vi "Custom Transient Response for Setpoints.vi"() -> (3 "SourceAdapt Parameters":T1 {"Current compensation frequency" scale=50.0..1000000.0 scale format="%#_6pHz"; "Voltage compensation frequency" scale=50.0..1000000.0 scale format="%#_6pHz"; "Current pole-zero ratio" scale=0.0625..16.0; "Current gain bandwidth" scale=10.0..1000000.0 scale format="%#_6pHz"; "Voltage pole-zero ratio" scale=0.0625..16.0; "Voltage gain bandwidth" scale=10.0..1000000.0 scale format="%#_6pHz"})   [LabVIEW 2021, in "PMIC Common.lvlib"]
uses:
  PMIC Common.lvlib
  controls/Multiple SourceAdapt Parameters.ctl
panel:
  in  "SingleSourceAdapt":string="Single SourceAdapt Parameters"
  in  "Multiple/Single SourceAdapt":bool=TRUE
  in  "Current":string="Current"
  in  "Voltage":string="Voltage"
  in  "Current compensation frequency":dbl(slide)=180000.0 caption="COMP. FREQUENCY" scale=50.0..1000000.0 scale format="%#_6pHz"
  in  "Voltage compensation frequency":dbl(slide)=3530.0 caption="COMP. FREQUENCY" scale=50.0..1000000.0 scale format="%#_6pHz"
  in  "Current pole-zero ratio":dbl(slide)=0.3 caption="POLE-ZERO RATIO" scale=0.0625..16.0
  in  "Current gain bandwidth":dbl(slide)=14000.0 caption="GAIN BANDWIDTH" scale=10.0..1000000.0 scale format="%#_6pHz"
  in  "Voltage pole-zero ratio":dbl(slide)=2.0 caption="POLE-ZERO RATIO" scale=0.0625..16.0
  in  "Voltage gain bandwidth":dbl(slide)=2000.0 caption="GAIN BANDWIDTH" scale=10.0..1000000.0 scale format="%#_6pHz"
  in  "SourceAdapt Parameters":T2(array[cluster]) {"Current compensation frequency" scale=50.0..1000000.0 scale format="%#_6pHz"; "Voltage compensation frequency" scale=50.0..1000000.0 scale format="%#_6pHz"; "Current pole-zero ratio" scale=0.0625..16.0; "Current gain bandwidth" scale=10.0..1000000.0 scale format="%#_6pHz"; "Voltage pole-zero ratio" scale=0.0625..16.0; "Voltage gain bandwidth" scale=10.0..1000000.0 scale format="%#_6pHz"}
  # "Voltage"
  # "Current"
  # "Voltage"
  # "Current"
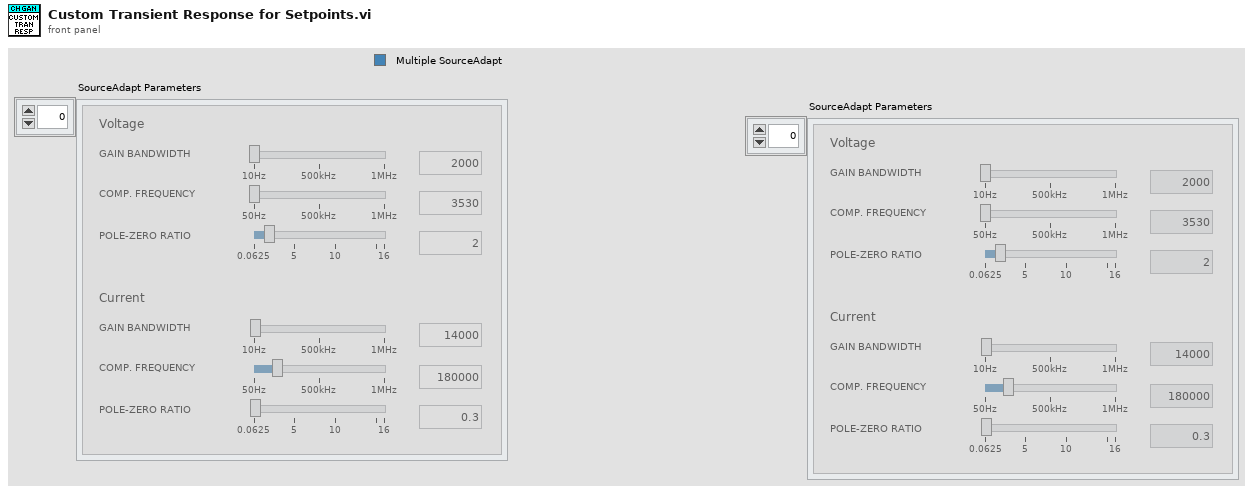
[diagram p1: front panel]
types:
  T1 = typedef "PMIC Common.lvlib/Multiple SourceAdapt Parameters.ctl" = cluster{"Voltage gain bandwidth":dbl, "Voltage compensation frequency":dbl, "Voltage pole-zero ratio":dbl, "Current gain bandwidth":dbl, "Current compensation frequency":dbl, "Current pole-zero ratio":dbl}[]
  T2 = cluster{"Voltage gain bandwidth":dbl, "Voltage compensation frequency":dbl, "Voltage pole-zero ratio":dbl, "Current gain bandwidth":dbl, "Current compensation frequency":dbl, "Current pole-zero ratio":dbl}[]
  T3 = enum32{"Invalid", "Standard", "Closed", "Hidden", "Minimized", "Maximized"}
  T4 = cluster{"Voltage gain bandwidth":dbl, "Voltage compensation frequency":dbl, "Voltage pole-zero ratio":dbl, "Current gain bandwidth":dbl, "Current compensation frequency":dbl, "Current pole-zero ratio":dbl}
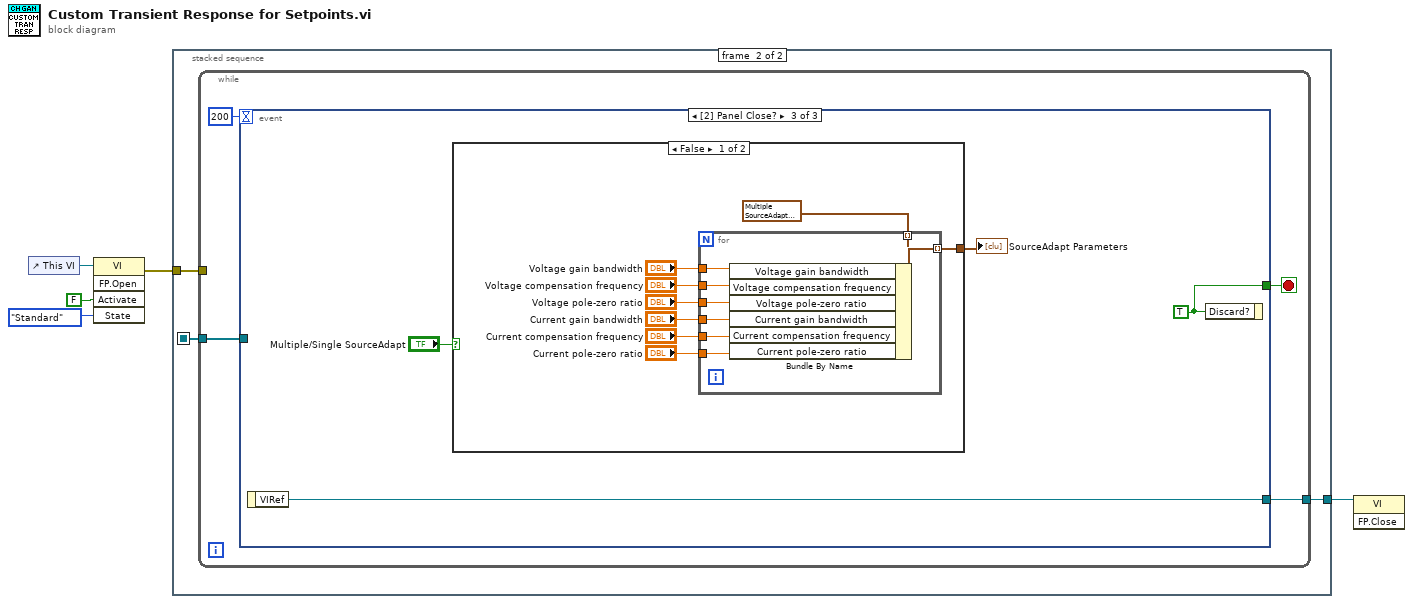
[diagram p0: block diagram]
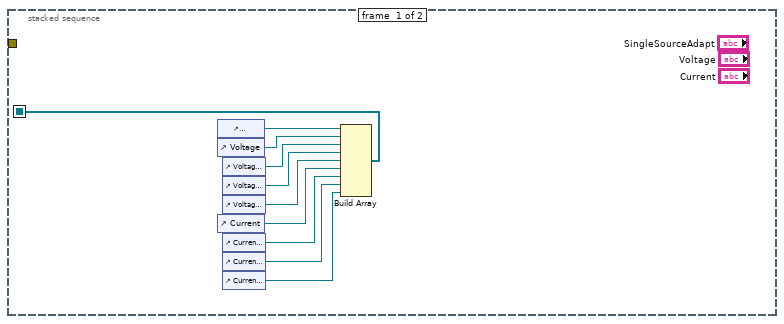
[diagram p2: hidden frame]
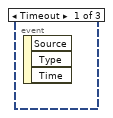
[diagram p3: hidden frame]
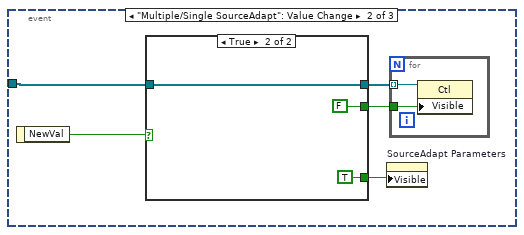
[diagram p4: hidden frame]
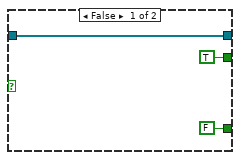
[diagram p5: hidden frame]
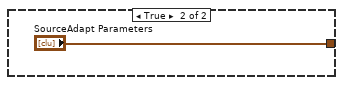
[diagram p6: hidden frame]
diagram:
  n1 = control-ref of="This VI"() -> (w5:refnum<vi>)
  n2 = invoke class="VI" method="FP.Open"(reference=w5, "Activate"=FALSE ("Activate?"), "State"=T3."Standard") -> (error out=w2:errorcluster)  [unwired: 2 in, 4 out]
  n3 = stacked-sequence {
    seq-local: [w9 _] -> [_ w16]
    tunnel: w2 -> [_ w18]
    tunnel: [_ w17] -> w1
    frame #0 {
      n4 = control-ref of="SingleSourceAdapt"() -> (w6:refnum<vi>)
      n5 = control-ref of="Voltage"() -> (w8:refnum<vi>)
      n6 = control-ref of="Current"() -> (w7:refnum<vi>)
      n7 = control-ref of="Voltage gain bandwidth"() -> (w15:refnum<vi>)
      n8 = control-ref of="Voltage compensation frequency"() -> (w14:refnum<vi>)
      n9 = control-ref of="Voltage pole-zero ratio"() -> (w13:refnum<vi>)
      n10 = control-ref of="Current gain bandwidth"() -> (w12:refnum<vi>)
      n11 = control-ref of="Current compensation frequency"() -> (w11:refnum<vi>)
      n12 = control-ref of="Current pole-zero ratio"() -> (w10:refnum<vi>)
      n13 = Build Array(w6, w8, w15, w14, w13, w7, w12, w11, w10) -> (w9:refnum<vi>[])
    }
    frame #1 {
      n14 = while {
        tunnel: [w20] -> w17
        tunnel: w18 -> [_]
        tunnel: w16 -> [w19]
        stop <- w22 stop-if-true
        n15 = event shown="[2] Panel Close?" {
          selector: _ -> [_ _ _]
          dyn-events: _ -> [_ _ _]
          timeout: 200 -> [_ _ _]
          tunnel: [_ _ w38] -> w22
          tunnel: [_ _ w39] -> w20
          tunnel: w19 -> [_ w23 _]
          event Timeout {
            n16 = event-data() -> ()  [unwired: 1 in, 3 out]
          }
          event "Multiple/Single SourceAdapt": Value Change {
            n17 = event-data() -> ("NewVal"=w27:bool)  [unwired: 1 in]
            n18 = case shown="True" w27 {
              tunnel: [TRUE ("Visible") FALSE ("Visible")] -> w26
              tunnel: [w30 w32] -> w25
              tunnel: w23 -> [w30 w32]
              tunnel: [FALSE ("Visible") TRUE ("Visible")] -> w24
              frame False {
              }
              frame True {
              }
            }
            n19 = property on="SourceAdapt Parameters" class="Arr (strict)"("Visible"=w24) -> ()  [unwired: 2 in, 2 out]
            n20 = for {
              tunnel: w26 -> [w35]
              tunnel: w25 -> [w34] mode=indexing
              n21 = property class="Ctl"(reference=w34, "Visible"=w35) -> ()  [unwired: 1 in, 2 out]
            }
          }
          event Panel Close? {
            w38 = TRUE ("Discard?")
            n22 = event-data() -> ("VIRef"=w39:refnum<vi>)  [unwired: 1 in]
            n23 = case shown="False" "Multiple/Single SourceAdapt" {
              tunnel: [w47 "SourceAdapt Parameters"] -> w36
              frame False {
                n24 = for {
                  tunnel: [w55] -> w47 mode=indexing
                  tunnel: T1 [{"Voltage gain bandwidth"=2000.0, "Voltage compensation frequency"=3530.0, "Voltage pole-zero ratio"=2.0, "Current gain bandwidth"=14000.0, "Current compensation frequency"=180000.0, "Current pole-zero ratio"=0.3}] -> [w54] mode=indexing
                  tunnel: "Voltage gain bandwidth" -> [w53]
                  tunnel: "Voltage compensation frequency" -> [w52]
                  tunnel: "Voltage pole-zero ratio" -> [w51]
                  tunnel: "Current gain bandwidth" -> [w50]
                  tunnel: "Current compensation frequency" -> [w49]
                  tunnel: "Current pole-zero ratio" -> [w48]
                  n25 = Bundle By Name(cluster=w54, "Voltage gain bandwidth"=w53, "Voltage compensation frequency"=w52, "Voltage pole-zero ratio"=w51, "Current gain bandwidth"=w50, "Current compensation frequency"=w49, "Current pole-zero ratio"=w48) -> (w55:T4)
                }
              }
              frame True {
              }
            }
            "SourceAdapt Parameters" <- w36
            n26 = event-data("Discard?"=w38) -> ()  [unwired: 1 in, 1 out]
          }
        }
      }
    }
  }
  n27 = invoke class="VI" method="FP.Close"(reference=w1) -> ()  [unwired: 2 in, 3 out]
